vi "TCP_Receiver_Main.vi"(8 "error in":errorcluster, 11 "Queue Ref":T1) -> (0 "error out":errorcluster)   [LabVIEW 2022 SP3]
uses:
  Controls/All Queue Ref.ctl
  Controls/TCP_Rec_Main.ctl
  Controls/ALL Health.ctl
  Loop.ctl
  6D_Global.vi
panel:
  out "Array":errorcluster[](array[cluster])
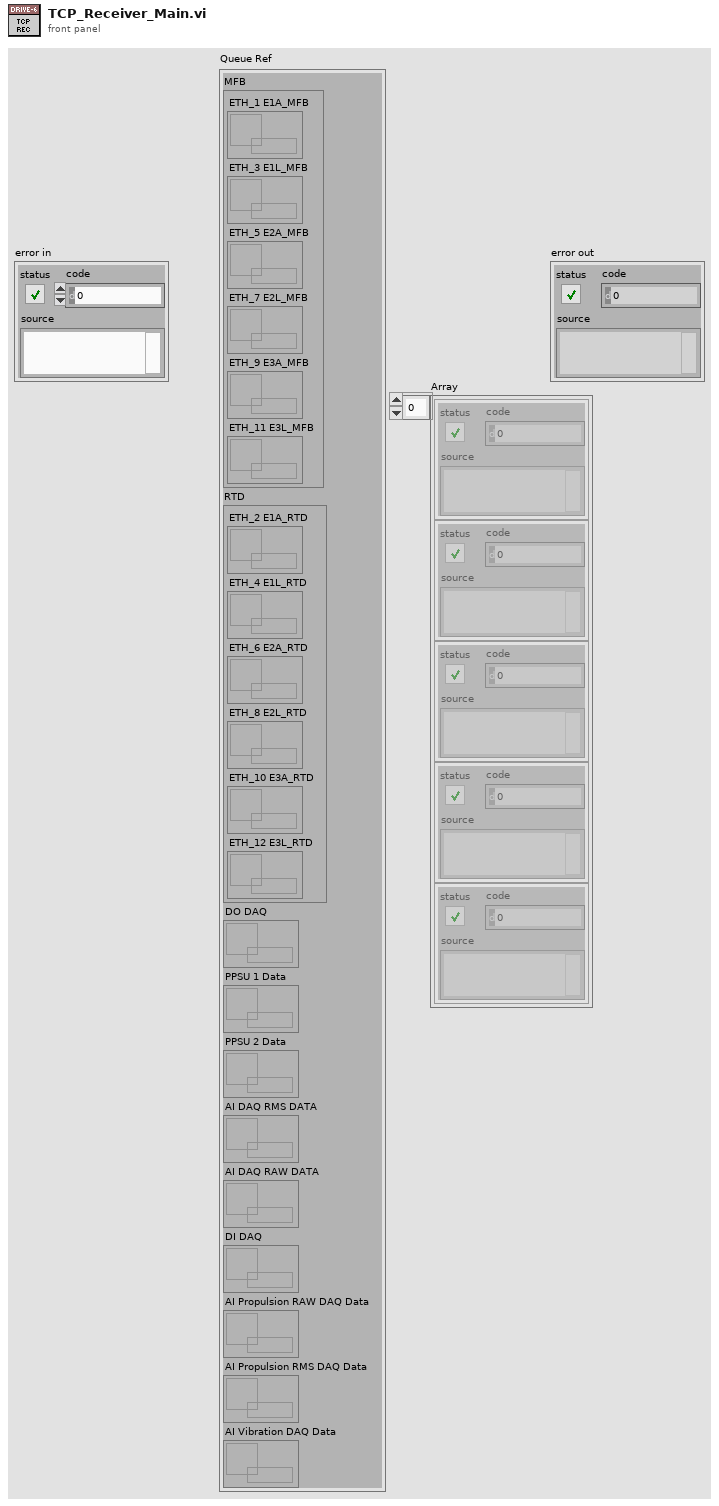
[diagram p1: front panel]
types:
  T1 = typedef "All Queue Ref.ctl" = cluster{"MFB":cluster{"ETH_1 E1A_MFB":refnum<queue>, "ETH_3 E1L_MFB":refnum<queue>, "ETH_5 E2A_MFB":refnum<queue>, "ETH_7 E2L_MFB":refnum<queue>, "ETH_9 E3A_MFB":refnum<queue>, "ETH_11 E3L_MFB":refnum<queue>}, "RTD":cluster{"ETH_2 E1A_RTD ":refnum<queue>, "ETH_4 E1L_RTD ":refnum<queue>, "ETH_6 E2A_RTD ":refnum<queue>, "ETH_8 E2L_RTD ":refnum<queue>, "ETH_10 E3A_RTD ":refnum<queue>, "ETH_12 E3L_RTD ":refnum<queue>}, "DO DAQ":refnum<queue>, "PPSU 1 Data":refnum<queue>, "PPSU 2 Data":refnum<queue>, "AI DAQ RMS DATA":refnum<queue>, "AI DAQ RAW DATA":refnum<queue>, "DI DAQ":refnum<queue>, "AI Propulsion RAW DAQ Data":refnum<queue>, "AI Propulsion RMS DAQ Data":refnum<queue>, "AI Vibration DAQ Data":refnum<queue>}
  T2 = cluster{"Listener ID":refnum<k5>[], "Bytes to read":i32[], "ETH_Names":string[], "Connect ID":refnum<k5>[], "Connected":string[], "Not Connected?":string[], "TCP Error":cluster{"TCP Error":refnum<k5>, "Error Chn":string}[], "in Progress?":bool, "GUI CMD ":cluster{"FC Command":cluster{"Size of Message":u8, "Primary Header":u8, "Secondary Header":u32, "Parameter ID":u8, "Parameter Data 1":u8, "Parameter ID 2":u8, "Parameter Data 2":u8}, "Com ON/OFF":bool[], "LCC ATS Hold":bool, "Start DAQ":bool, "Stop DAQ":bool, "RT EXIT":bool, "DO RT Array":bool[], "Initiate ALS":bool, "Upload to CRIO":bool[], "Download From CRIO":bool[], "Download From FC":bool[], "Upload to FC":bool[]}, "Buffered Bytes":i32[], "Numeric":u16, "Ports":u16[], "Wait on Listener":bool, "56,66 error":errorcluster[], "Queue Ref":T1}
  T3 = typedef "TCP_Rec_Main.ctl" = enum16{"Initialize", "Poll", "Receive Data", "Stop Server", "Exit", "Error"}
  T4 = enum16{"Init", "Read 'All'", "Read 'n'", "Read '1'", "Write '1'", "Write 'n'", "Write 'All'"}
  T5 = enum16{"Standard", "Buffered", "CRLF", "Immediate"}
  T6 = cluster{"Bytes to read":i32[], "ETH Names":string[], "Listener ID":refnum<k5>[], "Buffered Bytes":i32[], "Ports":u16[]}
  T7 = typedef "ALL Health.ctl" = enum16{"AI HS", "AI Vibration HS", "AI Propulsion HS", "DO HS", "Datalog HS", "PPSU HS", "ETH_1 DAQ", "ETH_1 RTD", "ETH_2 DAQ", "ETH_2 RTD", "ETH_5 RTD"}
  T8 = cluster{"ETH_1":bool, "ETH_2":bool, "ETH_3":bool, "ETH_4":bool, "ETH_5":bool}
  T9 = typedef "Loop.ctl" = enum16{"ETH_1", "ETH_2", "ETH_3", "ETH_4", "ETH_5", "ETH_6", "ETH_7", "ETH_8", "ETH_9", "ETH_10", "ETH_11", "ETH_12"}
  T10 = cluster{"TCP Error":refnum<k5>, "Error Chn":string}[]
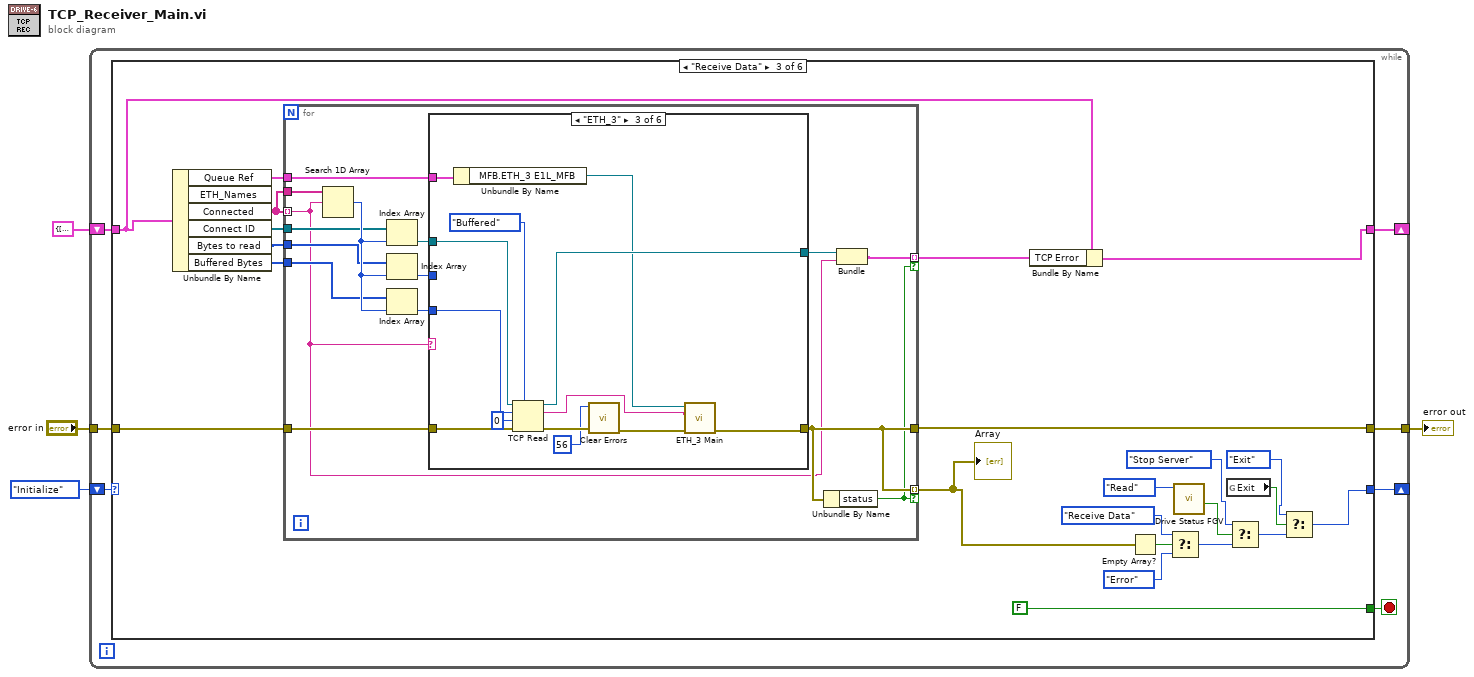
[diagram p0: block diagram]
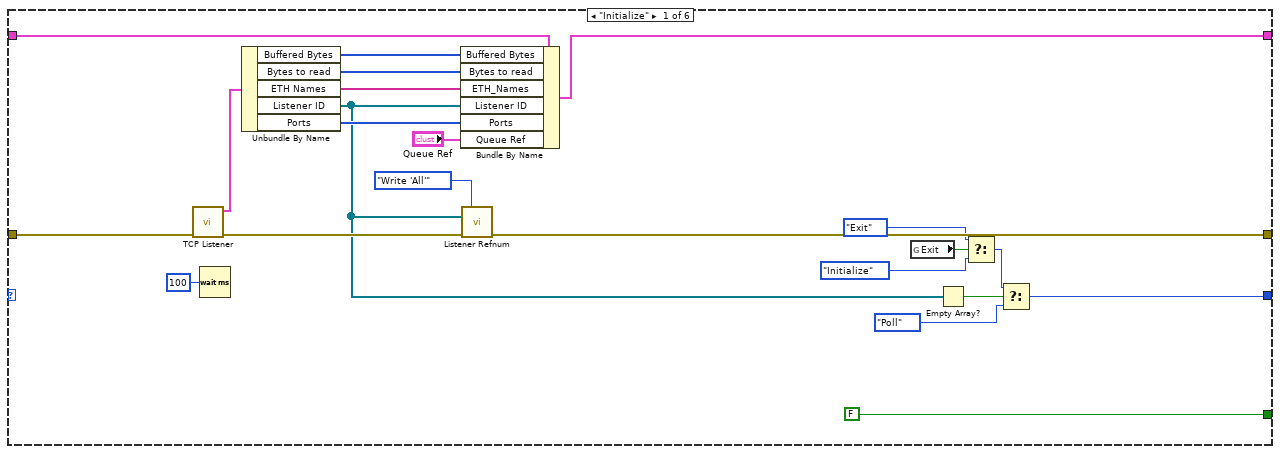
[diagram p2: hidden frame]
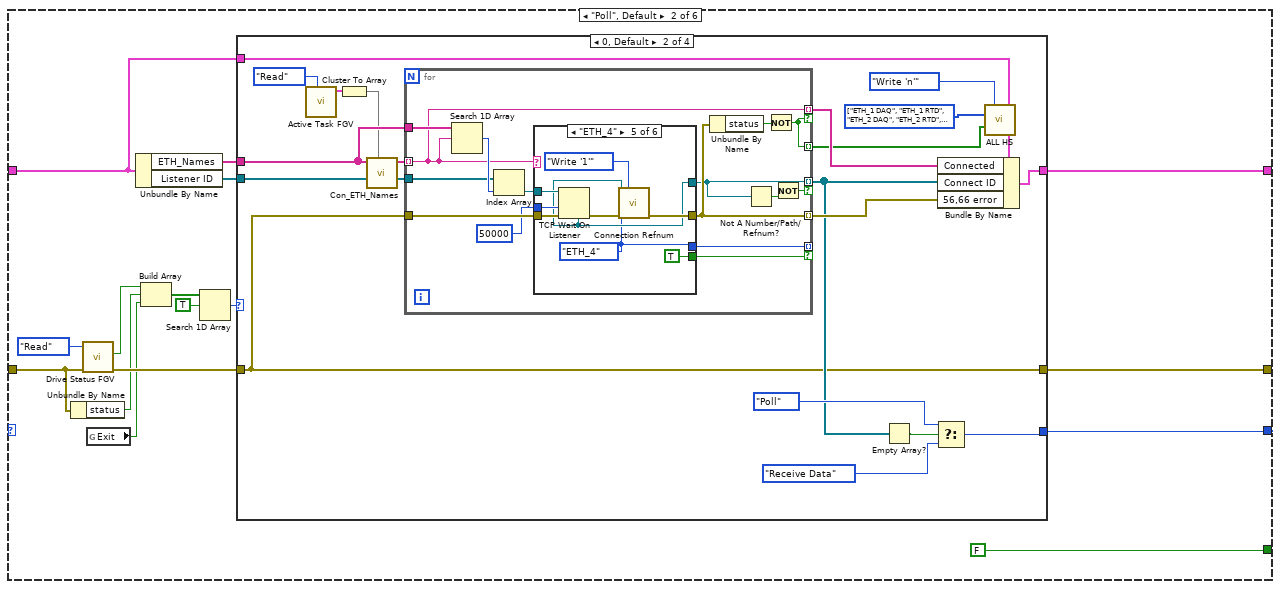
[diagram p3: hidden frame]
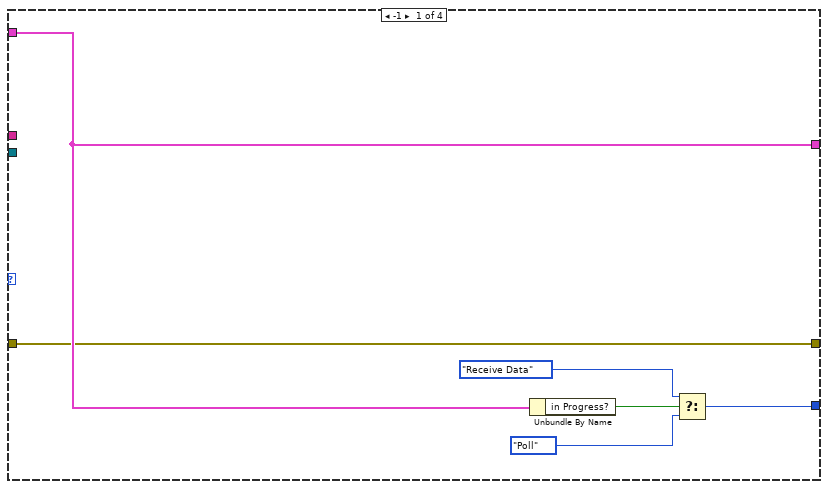
[diagram p4: hidden frame]
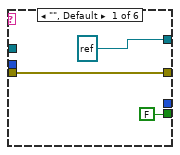
[diagram p5: hidden frame]
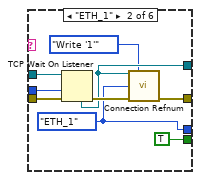
[diagram p6: hidden frame]
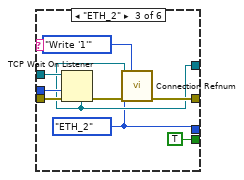
[diagram p7: hidden frame]
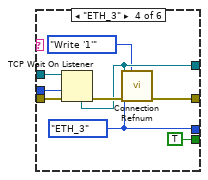
[diagram p8: hidden frame]
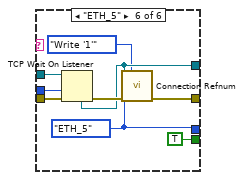
[diagram p9: hidden frame]
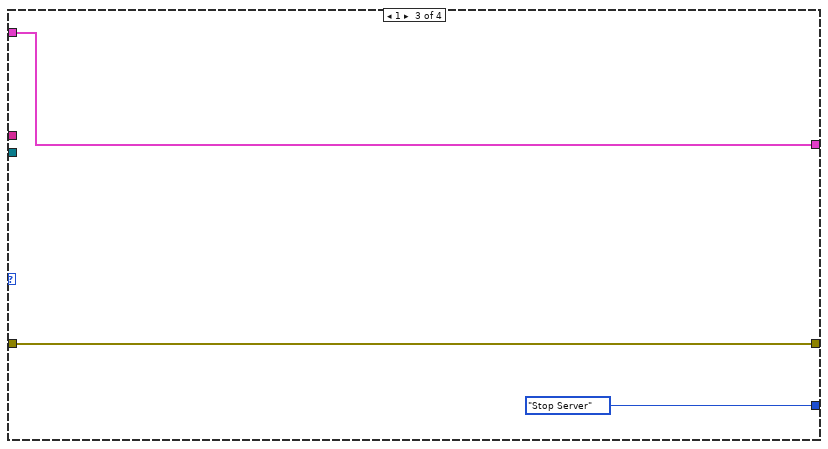
[diagram p10: hidden frame]
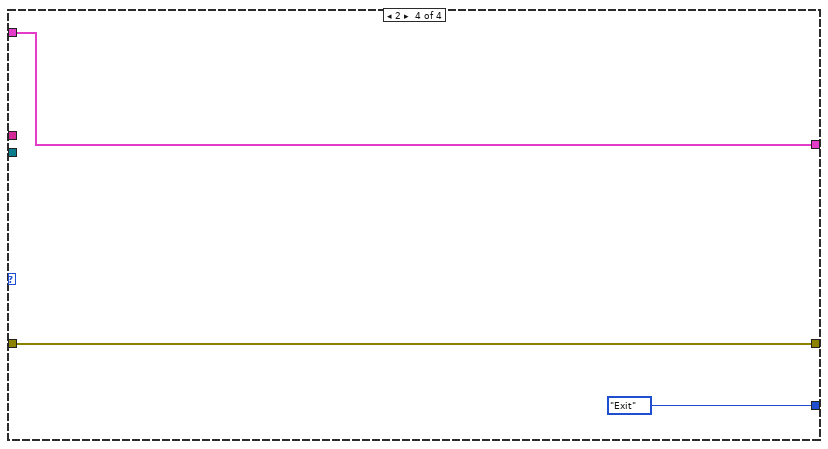
[diagram p11: hidden frame]
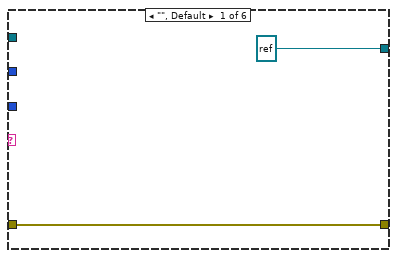
[diagram p12: hidden frame]
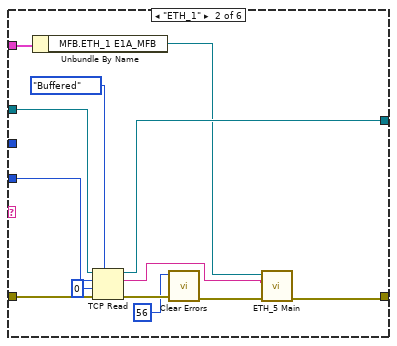
[diagram p13: hidden frame]
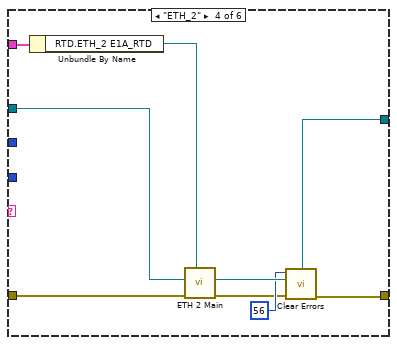
[diagram p14: hidden frame]
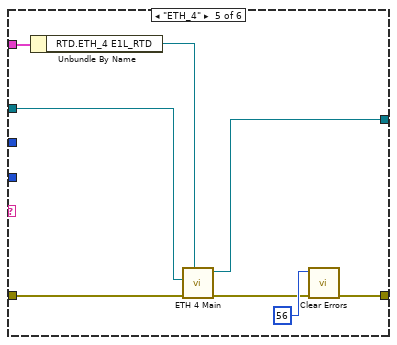
[diagram p15: hidden frame]
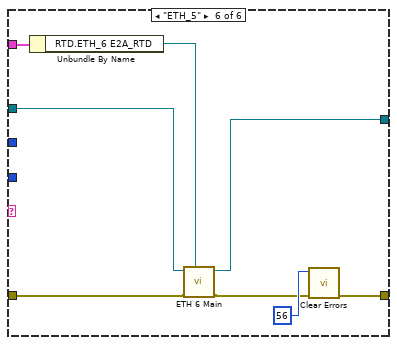
[diagram p16: hidden frame]
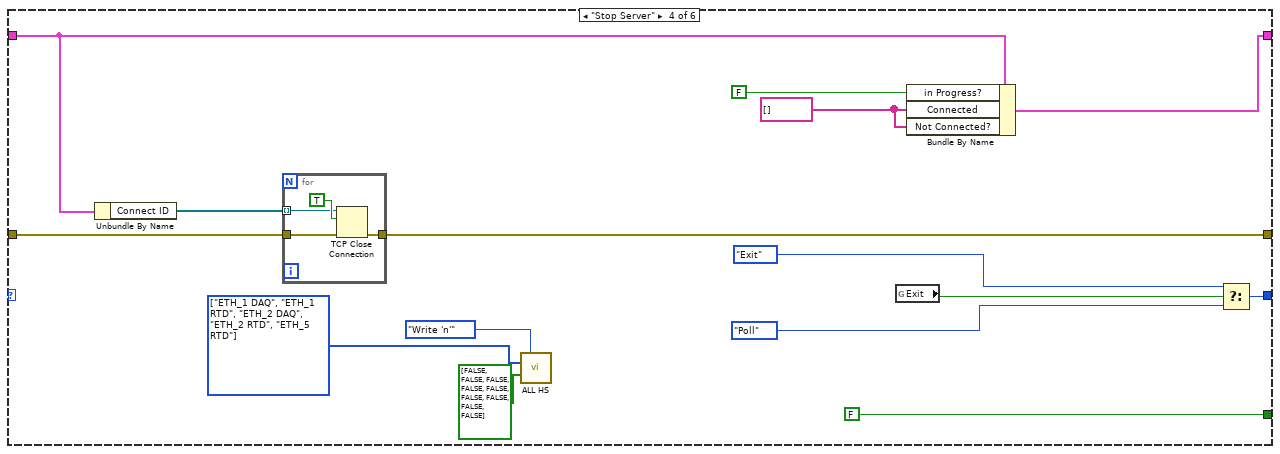
[diagram p17: hidden frame]
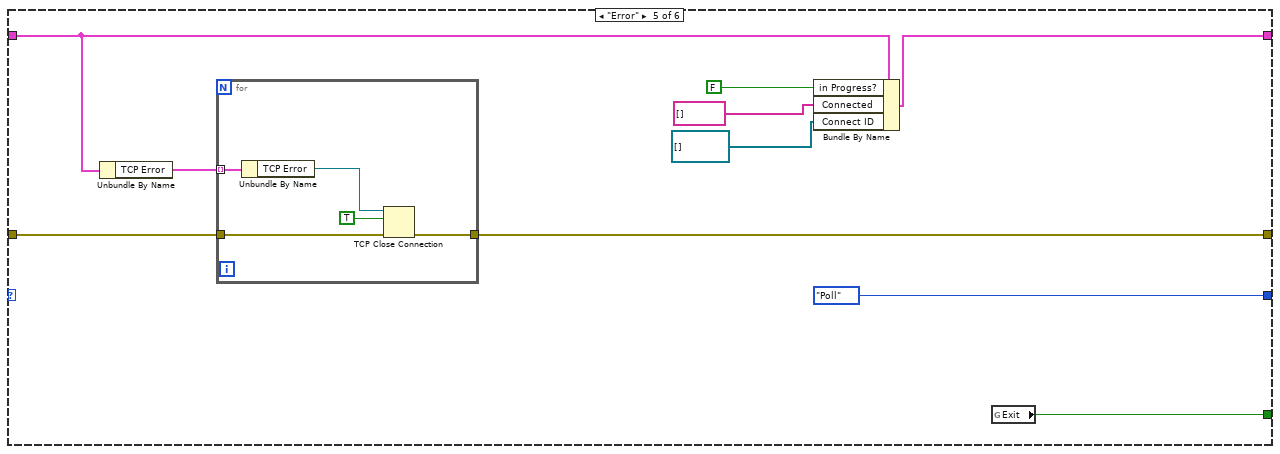
[diagram p18: hidden frame]
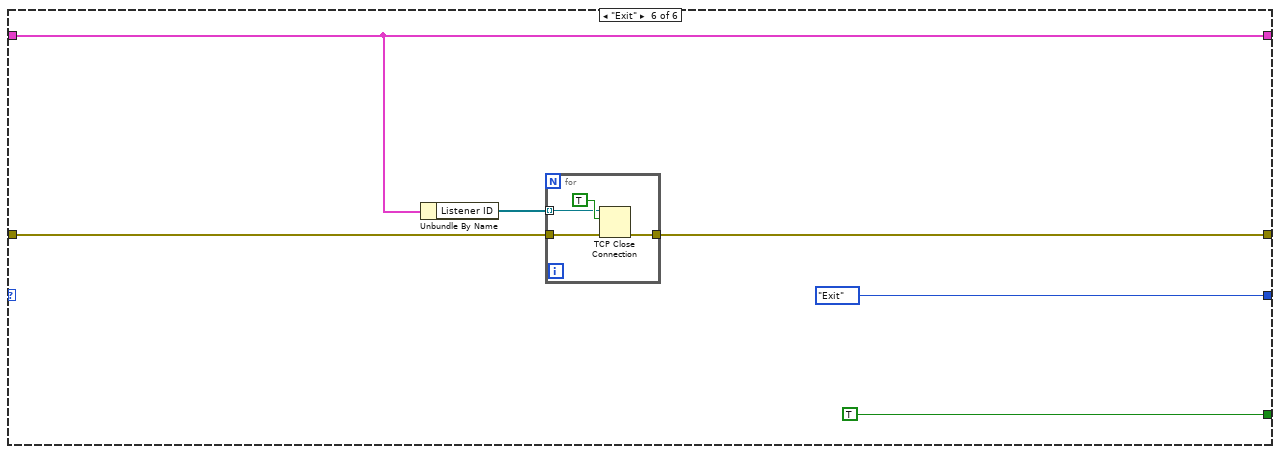
[diagram p19: hidden frame]
diagram:
  n1 = while {
    shift-right: [w8] -> _
    shift-left: TCP_Rec_Main."Initialize" -> [w11]
    tunnel: "error in" -> [w10]
    shift-right: [w7] -> _
    shift-left: T2 {"Listener ID"=[], "Bytes to read"=[], "ETH_Names"=[], "Connect ID"=[], "Connected"=[], "Not Connected?"=[], "TCP Error"=[], "in Progress?"=FALSE, "GUI CMD "={"FC Command"={"Size of Message"=0, "Primary Header"=0, "Secondary Header"=0, "Parameter ID"=0, "Parameter Data 1"=0, "Parameter ID 2"=0, "Parameter Data 2"=0}, "Com ON/OFF"=[], "LCC ATS Hold"=FALSE, "Start DAQ"=FALSE, "Stop DAQ"=FALSE, "RT EXIT"=FALSE, "DO RT Array"=[], "Initiate ALS"=FALSE, "Upload to CRIO"=[], "Download From CRIO"=[], "Download From FC"=[], "Upload to FC"=[]}, "Buffered Bytes"=[], "Numeric"=0, "Ports"=[], "Wait on Listener"=FALSE, "56,66 error"=[], "Queue Ref"={"MFB"={"ETH_1 E1A_MFB"=refnum, "ETH_3 E1L_MFB"=refnum, "ETH_5 E2A_MFB"=refnum, "ETH_7 E2L_MFB"=refnum, "ETH_9 E3A_MFB"=refnum, "ETH_11 E3L_MFB"=refnum}, "RTD"={"ETH_2 E1A_RTD "=refnum, "ETH_4 E1L_RTD "=refnum, "ETH_6 E2A_RTD "=refnum, "ETH_8 E2L_RTD "=refnum, "ETH_10 E3A_RTD "=refnum, "ETH_12 E3L_RTD "=refnum}, "DO DAQ"=refnum, "PPSU 1 Data"=refnum, "PPSU 2 Data"=refnum, "AI DAQ RMS DATA"=refnum, "AI DAQ RAW DATA"=refnum, "DI DAQ"=refnum, "AI Propulsion RAW DAQ Data"=refnum, "AI Propulsion RMS DAQ Data"=refnum, "AI Vibration DAQ Data"=refnum}} -> [w9]
    tunnel: [w6] -> w1
    stop <- w5 stop-if-true
    n2 = case shown="\"Receive Data\"" w11 {
      tunnel: w10 -> [w33 w39 w163 w244 w262 w270]
      tunnel: w9 -> [w31 w43 w162 w247 w258 w268]
      tunnel: [w21 w47 w144 w239 TCP_Rec_Main."Poll" TCP_Rec_Main."Exit"] -> w8
      tunnel: [w20 w42 w161 w246 w257 w268] -> w7
      tunnel: [w18 w40 w156 w243 w261 w271] -> w6
      tunnel: [FALSE FALSE FALSE FALSE w253 TRUE] -> w5
      frame "Initialize" {
        n3 = call "TCP Listener.vi"("error in"=w33) -> ("error out"=w26:errorcluster, "Port Config"=w32:T6)  [unwired: 9 in]
        n4 = Wait (ms)(milliseconds to wait=u32 100) -> ()  [unwired: 1 out]
        n5 = Unbundle By Name(w32) -> ("Buffered Bytes"=w30:i32[], "Bytes to read"=w29:i32[], "ETH Names"=w28:string[], "Listener ID"=w12:refnum<k5>[], "Ports"=w27:u16[])
        n6 = Bundle By Name(cluster=w31, "Buffered Bytes"=w30, "Bytes to read"=w29, "ETH_Names"=w28, "Listener ID"=w12, "Ports"=w27, "Queue Ref"="Queue Ref") -> (w20:T2)
        n7 = call "Listener Refnum.vi"("Option"=T4."Write 'All'", "Server  refnum"=w12, "error in"=w26) -> ("error out"=w18:errorcluster)  [unwired: 10 in, 2 out]
        n8 = global read "6D_Global.vi" "Exit"() -> (w15:bool)
        n9 = Empty Array?(array=w12) -> (empty?=w23:bool)
        n10 = Select(t=TCP_Rec_Main."Exit", s=w15, f=TCP_Rec_Main."Initialize") -> (s? t:f=w13:T3)
        n11 = Select(t=w13, s=w23, f=TCP_Rec_Main."Poll") -> (s? t:f=w21:T3)
      }
      frame "Poll", Default {
        n12 = Unbundle By Name(w39) -> ("status"=w38:bool)
        n13 = call "Drive Status FGV.vi"("error in"=w39, "Enum"=enum16{"Read", "Write"}."Read") -> ("error out"=w46:errorcluster, "Connect Drive Out"=w34:bool)  [unwired: 7 in, 1 out]
        n14 = global read "6D_Global.vi" "Exit"() -> (w35:bool)
        n15 = Unbundle By Name(w43) -> ("ETH_Names"=w45:string[], "Listener ID"=w44:refnum<k5>[])
        n16 = Build Array(w34, w38, w35) -> (w48:bool[])
        n17 = Search 1D Array(1D array=w48, element=TRUE) -> (index of element=w41:i32)  [unwired: 1 in]
        n18 = case shown="0, Default" w41 {
          tunnel: [w55 w69 TCP_Rec_Main."Stop Server" TCP_Rec_Main."Exit"] -> w47
          tunnel: w46 -> [w50 w62 w139 w142]
          tunnel: w45 -> [_ w73 _ _]
          tunnel: w44 -> [_ w72 _ _]
          tunnel: w43 -> [w52 w71 w140 w143]
          tunnel: [w52 w70 w140 w143] -> w42
          tunnel: [w50 w62 w139 w142] -> w40
          frame -1 {
            n19 = Unbundle By Name(w52) -> ("in Progress?"=w51:bool)
            n20 = Select(t=TCP_Rec_Main."Receive Data", s=w51, f=TCP_Rec_Main."Poll") -> (s? t:f=w55:T3)
          }
          frame 0, Default {
            w56 = T7[] [enum."ETH_1 DAQ", enum."ETH_1 RTD", enum."ETH_2 DAQ", enum."ETH_2 RTD", enum."ETH_5 RTD"] items=["AI HS", "AI Vibration HS", "AI Propulsion HS", "DO HS", "Datalog HS", "PPSU HS", "ETH_1 DAQ", "ETH_1 RTD", "ETH_2 DAQ", "ETH_2 RTD", "ETH_5 RTD"] ("Loops")
            n21 = call "Active Task FGV.vi"("Write/Read"=enum16{"Write", "Read"}."Read") -> ("Activate Task 2"=w58:T8)  [unwired: 9 in, 1 out]
            n22 = Cluster To Array(cluster=w58) -> (array=w57:bool[])
            n23 = call "Con_ETH_Names.vi"("Active ETH"=w57, "ETH_Names"=w73) -> ("To connect"=w74:string[])  [unwired: 8 in, 1 out]
            n24 = for {
              tunnel: w74 -> [w81] mode=indexing
              tunnel: w62 -> [w87]
              tunnel: w73 -> [w86]
              tunnel: w72 -> [w85]
              tunnel: [w78] -> w63 mode=indexing if=w75
              tunnel: [w83] -> w64 mode=indexing
              tunnel: [w81] -> w66 mode=indexing if=w76
              tunnel: [w80] -> _ mode=indexing if=w79
              tunnel: [w76] -> w59 mode=indexing
              n25 = Search 1D Array(1D array=w86, element=w81) -> (index of element=w88:i32)  [unwired: 1 in]
              n26 = Index Array(array=w85, index=w88) -> (element=w89:refnum<k5>)
              n27 = case shown="\"ETH_4\"" w81 {
                tunnel: w89 -> [_ w101 w110 w119 w128 w137]
                tunnel: w87 -> [w91 w100 w108 w117 w126 w135]
                tunnel: 50000 ("timeout ms (wait forever: -1)") -> [_ w99 w109 w118 w127 w136]
                tunnel: [refnum<k5> refnum ("listener ID") w95 w104 w113 w122 w131] -> w78
                tunnel: [w91 w97 w106 w115 w124 w133] -> w83
                tunnel: [_ w93 w102 w111 w120 w129] -> w80
                tunnel: [FALSE TRUE TRUE TRUE TRUE TRUE] -> w79
                frame "", Default {
                }
                frame "ETH_1" {
                  w93 = Loop."ETH_1" ("Loop")
                  n28 = TCP Wait On Listener(8:w100, 9:w99, 11:w101) -> (0:w98:errorcluster, 4:w95:refnum<k5>)  [unwired: 4 out]
                  n29 = call "Connection Refnum.vi"("ref"=w95, "Option"=T4."Write '1'", "Loop"=w93, "error in"=w98) -> ("error out"=w97:errorcluster)  [unwired: 9 in, 2 out]
                }
                frame "ETH_2" {
                  w102 = Loop."ETH_2" ("Loop")
                  n30 = TCP Wait On Listener(8:w108, 9:w109, 11:w110) -> (0:w107:errorcluster, 4:w104:refnum<k5>)  [unwired: 4 out]
                  n31 = call "Connection Refnum.vi"("ref"=w104, "Option"=T4."Write '1'", "Loop"=w102, "error in"=w107) -> ("error out"=w106:errorcluster)  [unwired: 9 in, 2 out]
                }
                frame "ETH_3" {
                  w111 = Loop."ETH_3" ("Loop")
                  n32 = TCP Wait On Listener(8:w117, 9:w118, 11:w119) -> (0:w116:errorcluster, 4:w113:refnum<k5>)  [unwired: 4 out]
                  n33 = call "Connection Refnum.vi"("ref"=w113, "Option"=T4."Write '1'", "Loop"=w111, "error in"=w116) -> ("error out"=w115:errorcluster)  [unwired: 9 in, 2 out]
                }
                frame "ETH_4" {
                  w120 = Loop."ETH_4" ("Loop")
                  n34 = TCP Wait On Listener(8:w126, 9:w127, 11:w128) -> (0:w125:errorcluster, 4:w122:refnum<k5>)  [unwired: 4 out]
                  n35 = call "Connection Refnum.vi"("ref"=w122, "Option"=T4."Write '1'", "Loop"=w120, "error in"=w125) -> ("error out"=w124:errorcluster)  [unwired: 9 in, 2 out]
                }
                frame "ETH_5" {
                  w129 = Loop."ETH_5" ("Loop")
                  n36 = TCP Wait On Listener(8:w135, 9:w136, 11:w137) -> (0:w134:errorcluster, 4:w131:refnum<k5>)  [unwired: 4 out]
                  n37 = call "Connection Refnum.vi"("ref"=w131, "Option"=T4."Write '1'", "Loop"=w129, "error in"=w134) -> ("error out"=w133:errorcluster)  [unwired: 9 in, 2 out]
                }
              }
              n38 = Unbundle By Name(w83) -> ("status"=w82:bool)
              n39 = Not A Number/Path/Refnum?(number/path/refnum=w78) -> (NaN/Path/Refnum?=w77:bool)
              n40 = Not(x=w82) -> (.not. x?=w76:bool)
              n41 = Not(x=w77) -> (.not. x?=w75:bool)
            }
            n42 = Empty Array?(array=w63) -> (empty?=w65:bool)
            n43 = Select(t=TCP_Rec_Main."Poll", s=w65, f=TCP_Rec_Main."Receive Data") -> (s? t:f=w69:T3)
            n44 = Bundle By Name(cluster=w71, "Connected"=w66, "Connect ID"=w63, "56,66 error"=w64) -> (w70:T2)
            n45 = call "ALL HS.vi"("Option"=T4."Write 'n'", "Loops"=w56, "Status List"=w59) -> ()  [unwired: 10 in, 3 out]
          }
          frame 1 {
          }
          frame 2 {
          }
        }
      }
      frame "Receive Data" {
        n46 = Unbundle By Name(w162) -> ("Queue Ref"=w158:T1, "Connected"=w157:string[], "Connect ID"=w166:refnum<k5>[], "Bytes to read"=w165:i32[], "Buffered Bytes"=w164:i32[])  [unwired: 1 out]
        n47 = for {
          tunnel: w157 -> [w170] mode=indexing
          tunnel: w166 -> [w180]
          tunnel: w165 -> [w179]
          tunnel: w164 -> [w178]
          tunnel: w163 -> [w174]
          tunnel: [w172] -> w145 mode=indexing if=w169
          tunnel: [w172] -> w156
          tunnel: [w171] -> w159 mode=indexing if=w169
          tunnel: w158 -> [w168]
          tunnel: w157 -> [w167]
          n48 = Search 1D Array(1D array=w167, element=w170) -> (index of element=w181:i32)  [unwired: 1 in]
          n49 = Index Array(array=w180, index=w181) -> (element=w177:refnum<k5>)
          n50 = Index Array(array=w179, index=w181) -> (element=w176:i32)
          n51 = Index Array(array=w178, index=w181) -> (element=w175:i32)
          n52 = case shown="\"ETH_3\"" w170 {
            tunnel: w177 -> [_ w195 w208 w214 w222 w227]
            tunnel: w176 -> [_ _ _ _ _ _]
            tunnel: w175 -> [_ w185 w202 _ _ _]
            tunnel: w174 -> [w183 w196 w209 w217 w225 w230]
            tunnel: [w183 w189 w205 w211 w218 w231] -> w172
            tunnel: [refnum<k5> refnum ("listener ID") w194 w207 w213 w221 w226] -> w173
            tunnel: w168 -> [_ w193 w206 w216 w224 w233]
            frame "", Default {
            }
            frame "ETH_1" {
              n53 = Unbundle By Name(w193) -> ("MFB.ETH_1 E1A_MFB"=w188:refnum<queue>)
              n54 = TCP Read(connection ID=w195, bytes to read=w185, error in (no error)=w196, 7:T5."Buffered" ("mode (standard)"), 9:0 ("timeout ms (25000)")) -> (connection ID out=w194:refnum<k5>, data out=w187:string, error out=w192:errorcluster)
              n55 = call <vilib>:"Clear Errors.vi"("error in (no error)"=w192, "specific error code to clear (0: all)"=56) -> ("error out"=w190:errorcluster)  [unwired: 4 in, 1 out]
              n56 = call "ETH_5 Main.vi"("error in"=w190, "data in"=w187, "ETH5-Q"=w188) -> ("error out"=w189:errorcluster)  [unwired: 8 in]
            }
            frame "ETH_3" {
              n57 = Unbundle By Name(w206) -> ("MFB.ETH_3 E1L_MFB"=w204:refnum<queue>)
              n58 = TCP Read(connection ID=w208, bytes to read=w202, error in (no error)=w209, 7:T5."Buffered" ("mode (standard)"), 9:0 ("timeout ms (25000)")) -> (connection ID out=w207:refnum<k5>, data out=w198:string, error out=w201:errorcluster)
              n59 = call <vilib>:"Clear Errors.vi"("error in (no error)"=w201, "specific error code to clear (0: all)"=56) -> ("error out"=w199:errorcluster)  [unwired: 4 in, 1 out]
              n60 = call "ETH_3 Main.vi"("error in"=w199, "data in"=w198, "ETH3-Q"=w204) -> ("error out"=w205:errorcluster)  [unwired: 8 in]
            }
            frame "ETH_2" {
              n61 = Unbundle By Name(w216) -> ("RTD.ETH_2 E1A_RTD"=w215:refnum<queue>)
              n62 = call "ETH 2 Main.vi"("ETH2 Q"=w215, "error in"=w217, "connection ID"=w214) -> ("error out"=w210:errorcluster, "connection ID 2"=w213:refnum<k5>)  [unwired: 7 in]
              n63 = call <vilib>:"Clear Errors.vi"("error in (no error)"=w210, "specific error code to clear (0: all)"=56) -> ("error out"=w211:errorcluster)  [unwired: 4 in, 1 out]
            }
            frame "ETH_4" {
              n64 = Unbundle By Name(w224) -> ("RTD.ETH_4 E1L_RTD"=w223:refnum<queue>)
              n65 = call "ETH 4 Main.vi"("ETH4 Q"=w223, "error in (no error)"=w225, "connection ID"=w222) -> ("error out 2"=w219:errorcluster, "connection ID 2"=w221:refnum<k5>)  [unwired: 7 in]
              n66 = call <vilib>:"Clear Errors.vi"("error in (no error)"=w219, "specific error code to clear (0: all)"=56) -> ("error out"=w218:errorcluster)  [unwired: 4 in, 1 out]
            }
            frame "ETH_5" {
              n67 = Unbundle By Name(w233) -> ("RTD.ETH_6 E2A_RTD"=w228:refnum<queue>)
              n68 = call "ETH 6 Main.vi"("ETH6 Q"=w228, "error in (no error)"=w230, "connection ID"=w227) -> ("error out 2"=w229:errorcluster, "connection ID 2"=w226:refnum<k5>)  [unwired: 7 in]
              n69 = call <vilib>:"Clear Errors.vi"("error in (no error)"=w229, "specific error code to clear (0: all)"=56) -> ("error out"=w231:errorcluster)  [unwired: 4 in, 1 out]
            }
          }
          n70 = Unbundle By Name(w172) -> ("status"=w169:bool)
          n71 = Bundle("connection ID 2"=w173, w170) -> (w171:cluster{"connection ID 2":refnum<k5>, string})  [unwired: 1 in]
        }
        "Array" <- w145
        n72 = Bundle By Name(cluster=w162, "TCP Error"=w159) -> (w161:T2)
        n73 = Empty Array?(array=w145) -> (empty?=w151:bool)
        n74 = Select(t=TCP_Rec_Main."Receive Data", s=w151, f=TCP_Rec_Main."Error") -> (s? t:f=w153:T3)
        n75 = call "Drive Status FGV.vi"("Enum"=enum16{"Read", "Write"}."Read") -> ("Disconnect Drive out"=w155:bool)  [unwired: 8 in, 2 out]
        n76 = global read "6D_Global.vi" "Exit"() -> (w152:bool)
        n77 = Select(t=TCP_Rec_Main."Stop Server", s=w155, f=w153) -> (s? t:f=w154:T3)
        n78 = Select(t=TCP_Rec_Main."Exit", s=w152, f=w154) -> (s? t:f=w144:T3)
      }
      frame "Stop Server" {
        w235 = T7[] [enum."ETH_1 DAQ", enum."ETH_1 RTD", enum."ETH_2 DAQ", enum."ETH_2 RTD", enum."ETH_5 RTD"] items=["AI HS", "AI Vibration HS", "AI Propulsion HS", "DO HS", "Datalog HS", "PPSU HS", "ETH_1 DAQ", "ETH_1 RTD", "ETH_2 DAQ", "ETH_2 RTD", "ETH_5 RTD"] ("Loops")
        w237 = string[] [] ("Connected")
        n79 = Unbundle By Name(w247) -> ("Connect ID"=w248:refnum<k5>[])
        n80 = for {
          tunnel: w248 -> [w251] mode=indexing
          tunnel: w244 -> [w250]
          tunnel: [w249] -> w243
          n81 = TCP Close Connection(connection ID=w251, abort (F)=TRUE, error in (no error)=w250) -> (error out=w249:errorcluster)  [unwired: 1 out]
        }
        n82 = call "ALL HS.vi"("Option"=T4."Write 'n'", "Loops"=w235, "Status List"=bool[] [FALSE, FALSE, FALSE, FALSE, FALSE, FALSE, FALSE, FALSE, FALSE]) -> ()  [unwired: 10 in, 3 out]
        n83 = global read "6D_Global.vi" "Exit"() -> (w242:bool)
        n84 = Bundle By Name(cluster=w247, "in Progress?"=FALSE, "Connected"=w237, "Not Connected?"=w237) -> (w246:T2)
        n85 = Select(t=TCP_Rec_Main."Exit", s=w242, f=TCP_Rec_Main."Poll") -> (s? t:f=w239:T3)
      }
      frame "Error" {
        n86 = Unbundle By Name(w258) -> ("TCP Error"=w259:T10)
        n87 = for {
          tunnel: w262 -> [w266]
          tunnel: [w265] -> w261
          tunnel: w259 -> [w264] mode=indexing
          n88 = Unbundle By Name(w264) -> ("TCP Error"=w263:refnum<k5>)
          n89 = TCP Close Connection(connection ID=w263, abort (F)=TRUE, error in (no error)=w266) -> (error out=w265:errorcluster)  [unwired: 1 out]
        }
        n90 = Bundle By Name(cluster=w258, "in Progress?"=FALSE, "Connected"=string[] [], "Connect ID"=refnum<k5>[] []) -> (w257:T2)
        n91 = global read "6D_Global.vi" "Exit"() -> (w253:bool)
      }
      frame "Exit" {
        n92 = Unbundle By Name(w268) -> ("Listener ID"=w269:refnum<k5>[])
        n93 = for {
          tunnel: w269 -> [w276] mode=indexing
          tunnel: w270 -> [w275]
          tunnel: [w274] -> w271
          n94 = TCP Close Connection(connection ID=w276, abort (F)=TRUE, error in (no error)=w275) -> (error out=w274:errorcluster)  [unwired: 1 out]
        }
      }
    }
  }
  "error out" <- w1
